vi "Get Size of Data from TD - Set Collection (1 String) - Returns Correct Size.vi"() -> ()   [LabVIEW 2017, in "Composition.Tests.lvlib"]
uses:
  Composition.Tests.lvlib
  <vilib>/addons/_JKI Toolkits/Caraya/classes/Assert/Assert Equal Value_Variant.vi
  Composition/Composition.lvlib
  <vilib>/addons/_JKI Toolkits/Caraya/classes/Assert/Assert.lvclass
  <vilib>/addons/_JKI Toolkits/Caraya/classes/Test/Test.lvclass
panel:
  out "error out":errorcluster
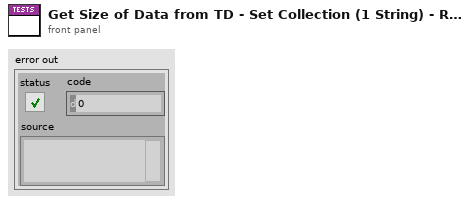
[diagram p1: front panel]
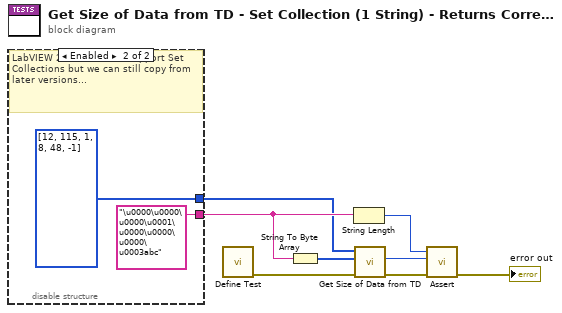
[diagram p0: block diagram]
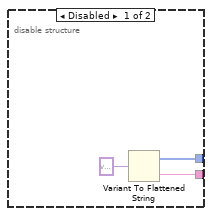
[diagram p2: hidden frame]
diagram:
  n1 = disable-structure shown="Enabled" {
    disable-tunnel: [w11 "\u0000\u0000\u0000\u0001\u0000\u0000\u0000\u0003abc" ("data string")] -> w7
    disable-tunnel: [w9 i16[] [12, 115, 1, 8, 48, -1] ("Type Descriptor")] -> w3
    frame Disabled {
      n2 = Variant To Flattened String(Variant=variant) -> (data string=w11:string, 1:w9:i16[])
    }
    frame Enabled {
      # "LabVIEW 2017 does not support Set Collections but we can still copy from later versions..."
    }
  }
  n3 = call <vilib>:"Define Test.vi"() -> ("error out"=w4:errorcluster)  [unwired: 11 in]
  n4 = String To Byte Array(string=w7) -> (unsigned byte array=w1:u8[])
  n5 = String Length(string=w7) -> (length=w5:i32)
  n6 = call "Get Size of Data from TD.vi"("error in (no error)"=w4, "Data String"=w1, "Type Descriptor"=w3) -> ("error out"=w8:errorcluster, "Size of Data"=w2:i32)  [unwired: 7 in]
  n7 = call-poly <vilib>:"Assert.vi"("error in (no error)"=w8, "Y"=w2, "X"=w5) -> ("error out"=→"error out":errorcluster)  [unwired: 8 in]
